vi "Add Remote Terminal.vi"(8 "error in":errorcluster, 10 "terminal address":u16, 11 "port in":T1 format="%.0x") -> (0 "error out":errorcluster, 2 "remote terminal":T1 format="%.0x", 3 "port out":T1 format="%.0x")   [LabVIEW 2020, in "Ballard MIL-STD-1553 Scripting.lvlib"]
uses:
  Ballard MIL-STD-1553 Scripting.lvlib
  <vilib>/NI VeriStand/Custom Device API/Custom Device Item Ref.ctl
  <vilib>/NI VeriStand/Custom Device API/Custom Device Channel.ctl
  <vilib>/NI VeriStand/Custom Device API/Custom Device Channel Type.ctl
  Constants.vi
  <vilib>/NI VeriStand/Custom Device API/Custom Device API.lvlib
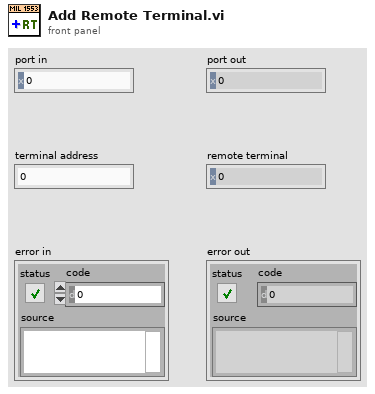
[diagram p1: front panel]
types:
  T1 = typedef "Custom Device API.lvlib/Custom Device Item Ref.ctl" = u64
  T2 = typedef "Custom Device API.lvlib/Custom Device Channel.ctl" = cluster{"Type":T3, "Units":string, "Default Value":dbl, "Faultable":bool, "Scalable":bool}
  T3 = typedef "Custom Device API.lvlib/Custom Device Channel Type.ctl" = enum16{"Input", "Output"}
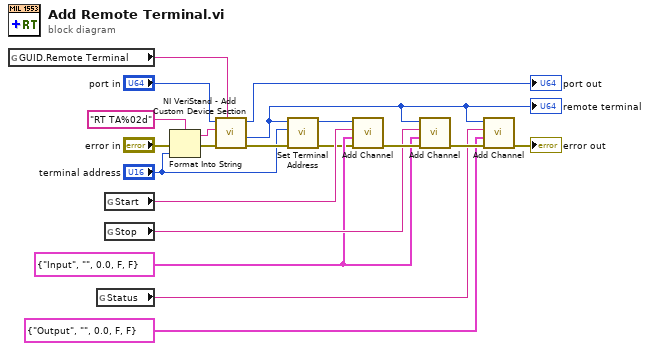
[diagram p0: block diagram]
diagram:
  w14 = T2 {"Type"=enum."Input", "Units"="", "Default Value"=0.0, "Faultable"=FALSE, "Scalable"=FALSE} ("Channel")
  n1 = global read "Constants.vi" "GUID.Remote Terminal"() -> (w20:string)
  n2 = global read "Constants.vi" "Status"() -> (w12:string)
  n3 = global read "Constants.vi" "Start"() -> (w16:string)
  n4 = global read "Constants.vi" "Stop"() -> (w15:string)
  n5 = Format Into String(format string="RT TA%02d", error in="error in", "terminal address") -> (resulting string=w3:string, error out=w1:errorcluster)  [unwired: 1 in]
  n6 = call <vilib>:"NI VeriStand - Add Custom Device Section.vi"("GUID (Default Section)"=w20, "error in (no error)"=w1, "Section Name"=w3, "Parent Ref in"="port in") -> ("error out"=w6:errorcluster, "Section Ptr"=w8:T1, "Parent Ref out"=→"port out":T1)  [unwired: 4 in, 1 out]
  "remote terminal" <- w8
  n7 = call "Set Terminal Address.vi"("error in"=w6, "terminal address"="terminal address", "remote terminal in"=w8) -> ("error out"=w5:errorcluster, "remote terminal out"=w7:T1)  [unwired: 7 in]
  n8 = call "Add Channel.vi"("error in"=w5, "Channel"=w14, "Name"=w16, "Frame Ref"=w7) -> ("error out"=w17:errorcluster)  [unwired: 6 in, 1 out]
  n9 = call "Add Channel.vi"("error in"=w17, "Channel"=w14, "Name"=w15, "Frame Ref"=w8) -> ("error out"=w13:errorcluster)  [unwired: 6 in, 1 out]
  n10 = call "Add Channel.vi"("error in"=w13, "Channel"=T2 {"Type"=enum."Output", "Units"="", "Default Value"=0.0, "Faultable"=FALSE, "Scalable"=FALSE}, "Name"=w12, "Frame Ref"=w8) -> ("error out"=→"error out":errorcluster)  [unwired: 6 in, 1 out]
